vi "ClassMethod.vi"(8 "error in (no error)":errorcluster, 11 "GCode_Parrent_Class in":refnum<class "GCode_Parrent_Class.lvclass">) -> (0 "error out":errorcluster, 3 "GCode_Parrent_Class out":refnum<class "GCode_Parrent_Class.lvclass">)   [LabVIEW 2014, in "GCode_Parrent_Class.lvclass"]
uses:
  GCode_Parrent_Class.lvclass
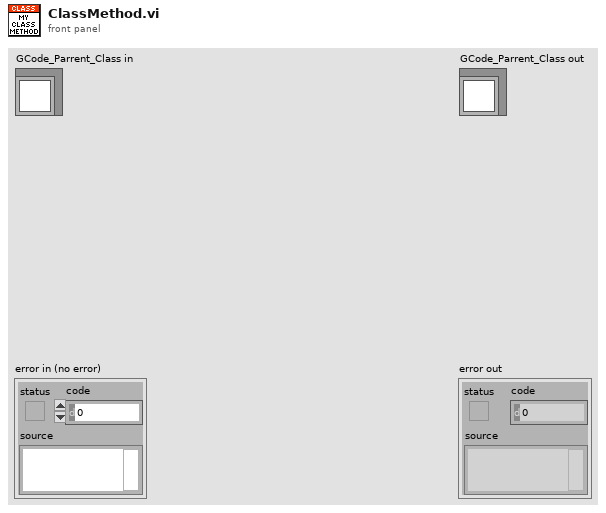
[diagram p1: front panel]
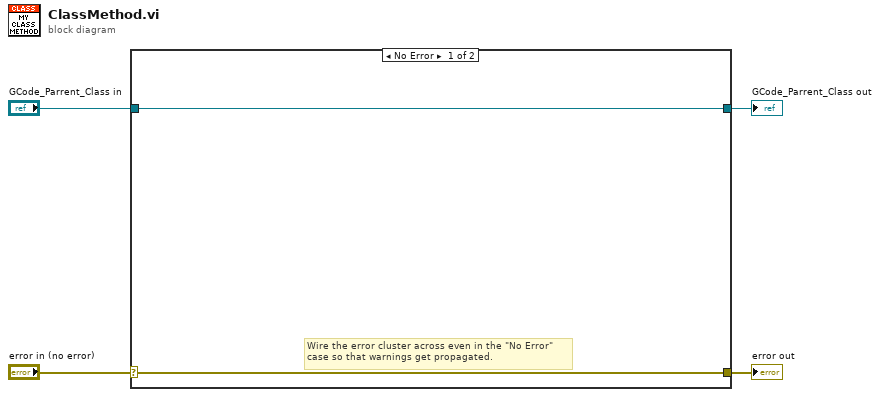
[diagram p0: block diagram]
diagram:
  n1 = case shown="No Error" "error in (no error)" {
    selector: "error in (no error)" -> [w5 w8]
    tunnel: [w5 w8] -> w3
    tunnel: [w6 w7] -> w1
    tunnel: "GCode_Parrent_Class in" -> [w6 w7]
    frame No Error {
      # "Wire the error cluster across even in the \"No Error\"\ncase so that warnings get propagated."
    }
    frame Error {
    }
  }
  "error out" <- w3
  "GCode_Parrent_Class out" <- w1
